vi "实时数据发送间隔全局.vi"() -> ()   [LabVIEW 2016, in "数据传输系统-06.lvlib"]
panel:
  in  "实时数据发送间隔":u32
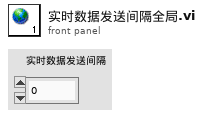
[diagram p1: front panel]
diagram:
